vi "ex7.vi"() -> ()   [LabVIEW 2022 SP3]
panel:
  in  "Reset Timer":bool caption="Reset"
  out "Elapsed time [ms]":dbl caption="Elapsed Time (s)"
  in  "?":bool
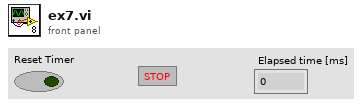
[diagram p1: front panel]
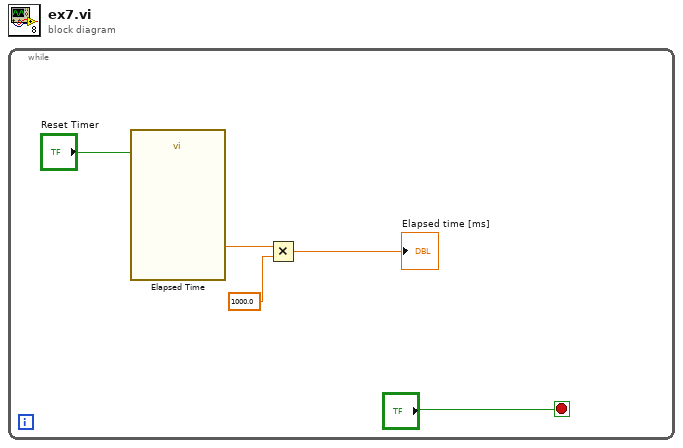
[diagram p0: block diagram]
diagram:
  n1 = while {
    stop <- "?" stop-if-true
    n2 = call "Elapsed Time"("Reset"="Reset Timer") -> ("Elapsed Time (s)"=w2:dbl)  [unwired: 11 in, 7 out]
    n3 = Multiply(x=w2, y=1000.0) -> (x*y=→"Elapsed time [ms]":dbl)
  }
